vi "ContextHelp_HelpTexts.vi"(0 "HelpText (enum or string)":variant) -> (14 "HelpOut":T2, 15 "NotFound":bool)   [LabVIEW 2014]
uses:
  <resource>/Framework/Providers/Open_GDS/UML/ContextHelp/ContextHelp_ShowType.ctl
  <resource>/Framework/Providers/Open_GDS/UML/ContextHelp/ContextHelp_HelpTexts.ctl
panel:
  in  "HelpText 2":T1
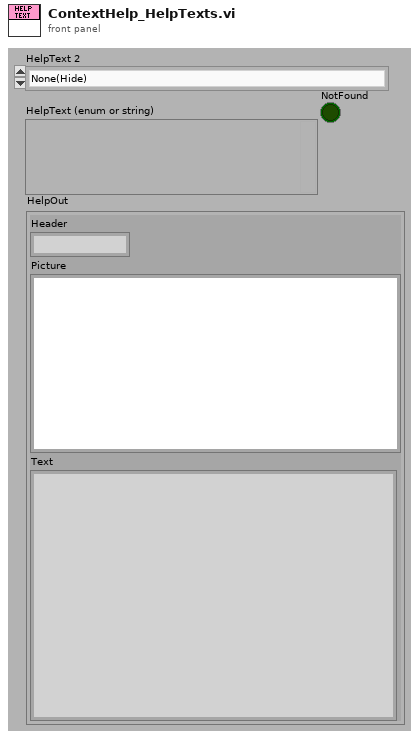
[diagram p1: front panel]
types:
  T1 = typedef "ContextHelp_HelpTexts.ctl" = enum16{"None(Hide)", "Default", "Help", "Welcome", "GettingStarted", "ClassDiagram_Help", "SequenceDiagram_Help", "UseCaseDiagram_Help", "BSelect", "BClass", "BInterface", "BPackage", "BNote", "BDependency", "BInheritance", "BInterfaceImplementation", "BAssociation", "BAggregation", "BCompAggregation", "BNoteConnector", "BObject", "BActionBar", "BCall", "BSystem", "BActor", "BUseCase", "BGeneralization", "BIncludes", "BExtends", "BUseCaseDiagramAssociation", "ClassRelationshipEdge editDialog_Bent Style", "ClassRelationshipEdge editDialog_RelationType", "ClassRelationshipEdge editDialog_Reverse association", "ClassRelationshipEdge editDialog_Start label", "ClassRelationshipEdge editDialog_Middle label", "ClassRelationshipEdge editDialog_End label", "UMLEditor reversedEngineering_Pathes", "ReversedEngineering StateReverseDialog_Help", "ReversedEngineering StateQueuedSettings_Help", "UMLEditor reversedEngineering_AddTopVIs", "UMLEditor reversedEngineering_AddClasses", "UMLEditor reversedEngineering_AddDirs", "UMLEditor reversedEngineering_Recursively", "UMLEditor reversedEngineering_Remove", "UMLEditor reversedEngineering_ClearList", "UMLEditor reversedEngineering_HideSubAss", "UMLEditor reversedEngineering_CreateTypes", "UMLEditor reversedEngineering_OnlyInheritance", "UMLEditor reversedEngineering_CreateApplication", "UMLEditor reversedEngineering_OK", "UMLEditor reversedEngineering_Cancel", "UMLEditor reversedEngineering_Help", "UMLEditor createWizardScriptFile_ScriptfilePath", "UMLEditor createWizardScriptFile_ClassPath", "UMLEditor createWizardScriptFile_Use", "UMLEditor createWizardScriptFile_PrivateDirName", "UMLEditor createWizardScriptFile_DirAppend", "UMLEditor createWizardScriptFile_Separator Character", "UMLEditor createWizardScriptFile_OK", "UMLEditor createWizardScriptFile_Cancel", "UMLEditor createWizardScriptFile_Help", "ClassNode editDialog_Class Name", "InterfaceNode editDialog_Class Name", "ClassNode editDialog_Attribute", "ClassNode editDialog_Methods", "InterfaceNode editDialog_Methods", "ClassNode editDialog_connection", "InterfaceNode editDialog_connection", "ClassNode editDialog_StereoType", "ClassNode editDialog_ShowAttrib", "ClassNode editDialog_ShowMethods", "ClassNode editDialog_ClassPath", "ClassNode editDialog_AddAttribute", "ClassNode editDialog_AddMethod", "InterfaceNode editDialog_AddMethod", "ClassNode AttributeGuide_AttributeName", "ClassNode AttributeGuide_Array?", "ClassNode AttributeGuide_Data Type", "ClassNode AttributeGuide_RefName", "ClassNode AttributeGuide_Preview", "ClassNode AttributeGuide_OK", "ClassNode AttributeGuide_Cancel", "ClassNode MethodGuide_Visibility", "ClassNode MethodGuide_Method Name", "ClassNode MethodGuide_Preview", "ClassNode MethodGuide_OK", "ClassNode MethodGuide_Cancel", "CallNode EditCallProperties_AllButtons", "ObjectNode EditObjectlProperties_AllButtons", "ActorNode EditActorProperties_AllButtons", "UseCaseRelationshipNode EditUseCaselProperties_AllButtons", "UseCaseNode EditUseCaselProperties_AllButtons", "SystemNode EditSystemProperties_AllButtons", "ReversedEngineering UpdateAttributes_AllButtons", "StateNode editDialog_AllButtons", "StateTransition editDialog_AllButtons", "ArrangeNodes Main_Picture", "ArrangeNodes Main_Zoom", "ArrangeNodes Main_Auto Zoom", "ArrangeNodes Main_shorten", "ArrangeNodes Main_Min Length", "ArrangeNodes Main_Max Length", "ArrangeNodes Main_increase", "ArrangeNodes Main_decrease", "ArrangeNodes Main_Shake", "ArrangeNodes Main", "BState", "BInitialState", "BFinalState", "BStateTransition", "StateDiagram_Help", "StateDiagram_PropertiesAllButtons", "ReversedEngineering StateReverseDialog_ClearStates", "ReversedEngineering StateReverseDialog_UseQueuedStateMachines", "ReversedEngineering StateReverseDialog_QueuedSettings", "ReversedEngineering StateReverseDialog_SearchForVIs", "ReversedEngineering StateReverseDialog_SearchCriteria", "OptionsDialog_ClassBasePath", "OptionsDialog_VIPath", "OptionsDialog_ApplicationPath", "OptionsDialog_WizDir", "OptionsDialog_IniFilePath", "OptionsDialog_DefineColors", "OptionsDialog_Help", "OptionsDialog_CreateTypes", "ClassRelationshipEdge editDialog_SplitWire"}
  T2 = typedef "ContextHelp_ShowType.ctl" = cluster{"Header":string, "Picture":picture, "Text":string}
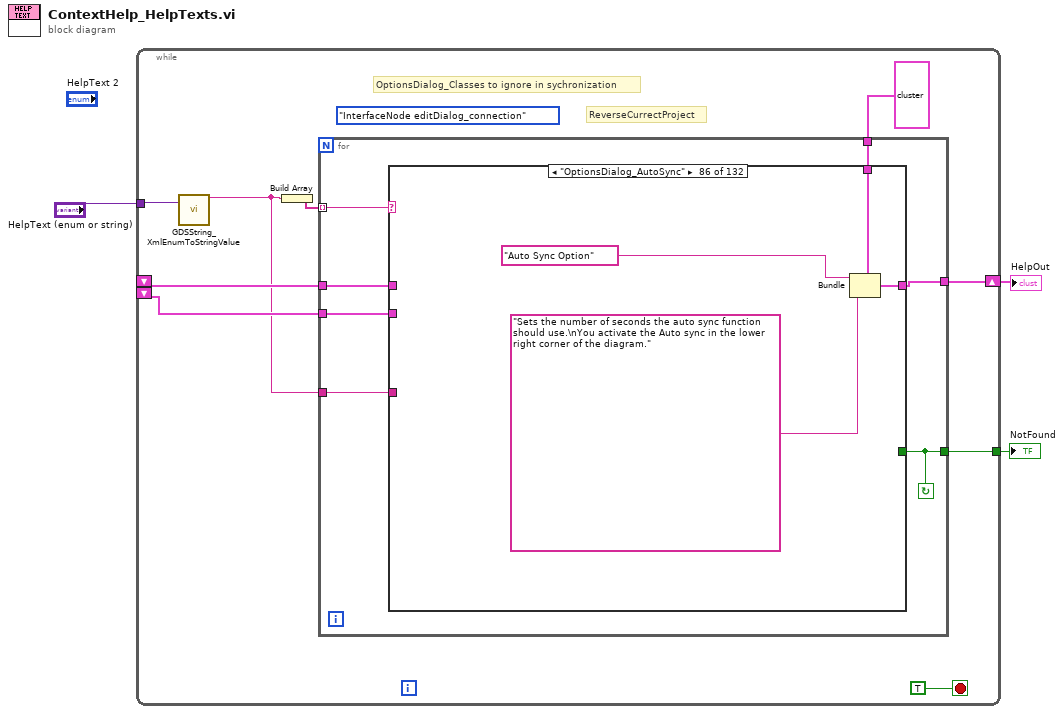
[diagram p0: block diagram]
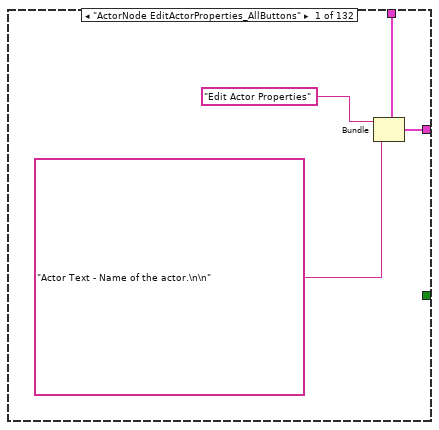
[diagram p2: hidden frame]
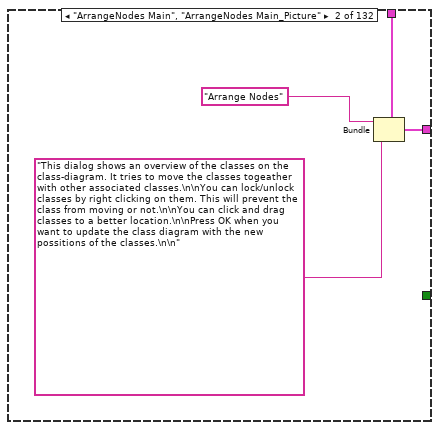
[diagram p3: hidden frame]
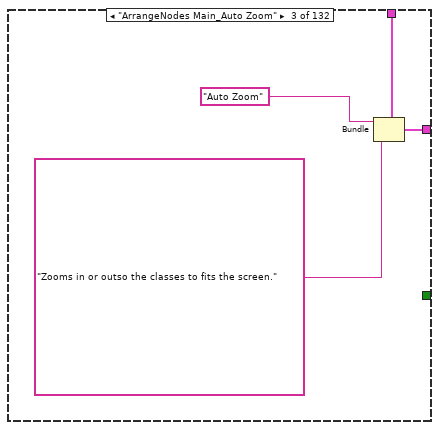
[diagram p4: hidden frame]
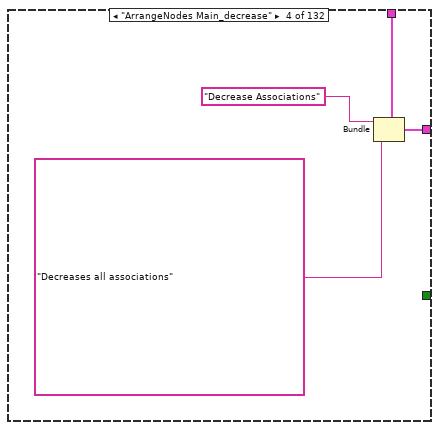
[diagram p5: hidden frame]
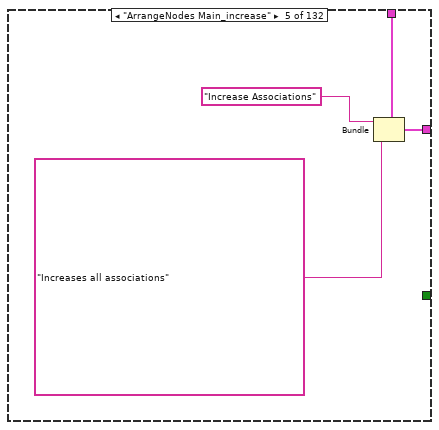
[diagram p6: hidden frame]
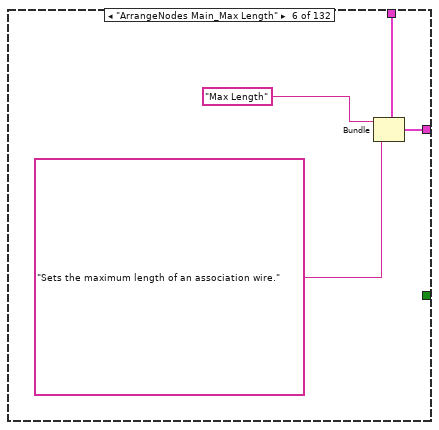
[diagram p7: hidden frame]
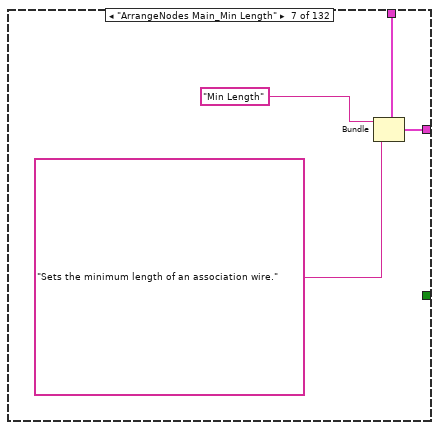
[diagram p8: hidden frame]
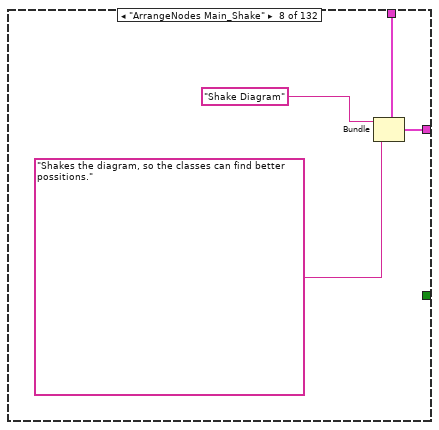
[diagram p9: hidden frame]
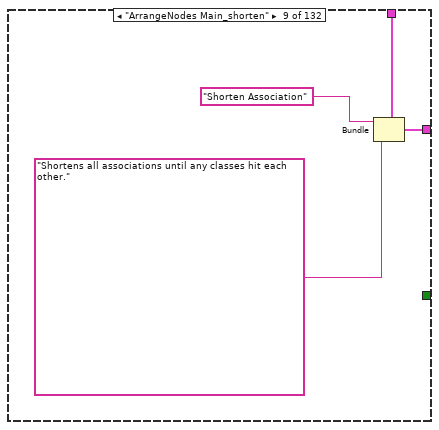
[diagram p10: hidden frame]
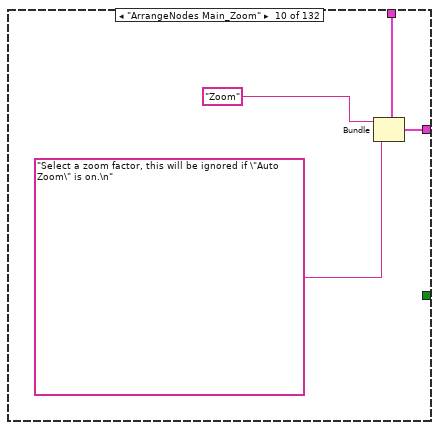
[diagram p11: hidden frame]
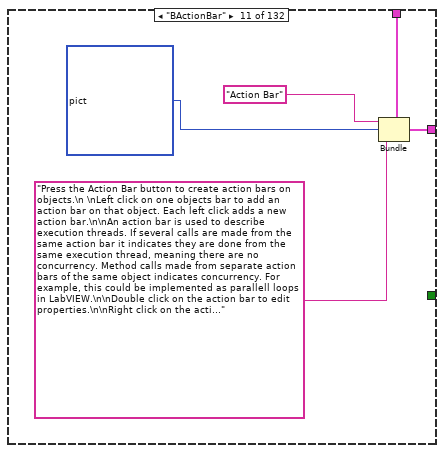
[diagram p12: hidden frame]
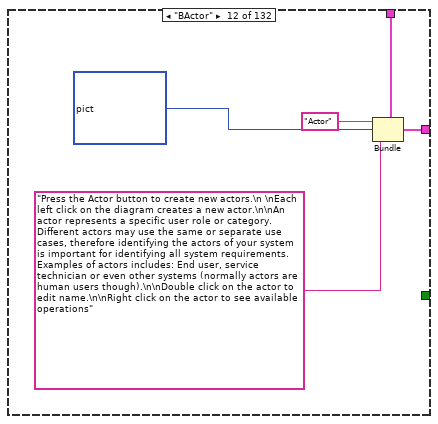
[diagram p13: hidden frame]
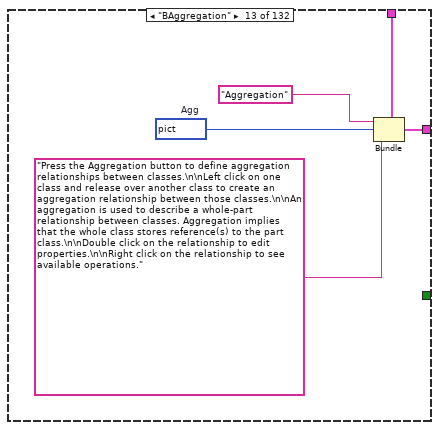
[diagram p14: hidden frame]
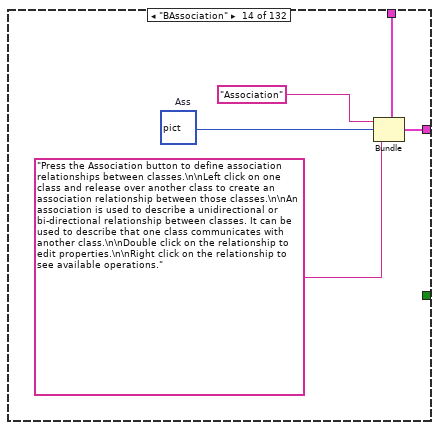
[diagram p15: hidden frame]
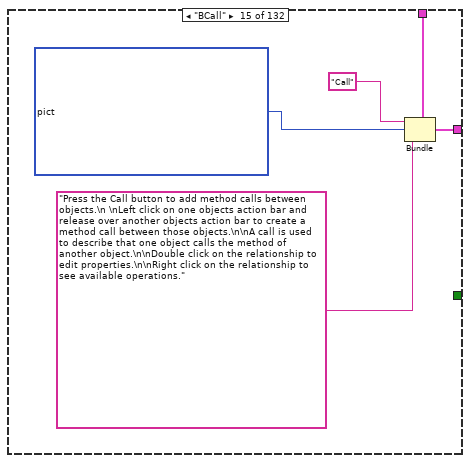
[diagram p16: hidden frame]
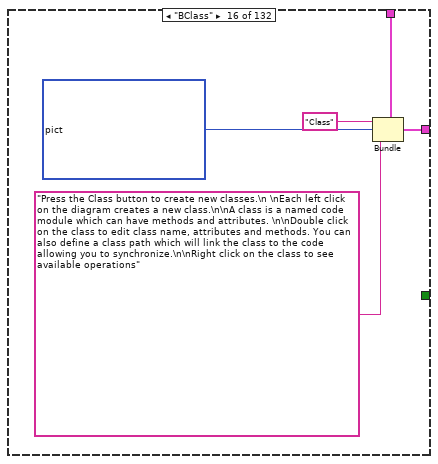
[diagram p17: hidden frame]
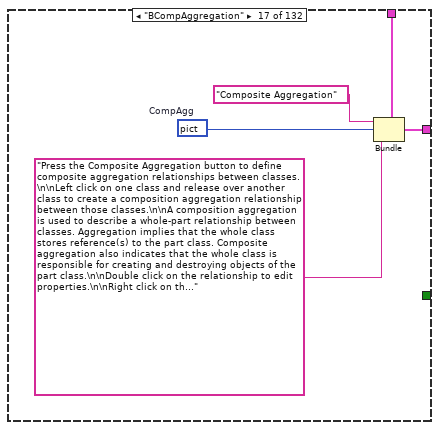
[diagram p18: hidden frame]
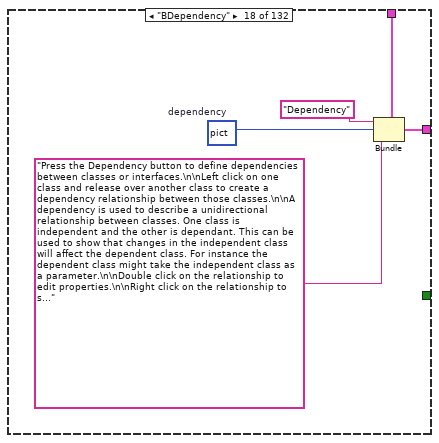
[diagram p19: hidden frame]
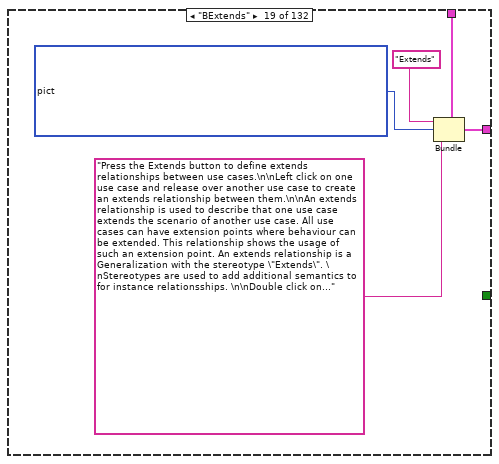
[diagram p20: hidden frame]
diagram:
  n1 = while {
    tunnel: "HelpText (enum or string)" -> [w7]
    shift-right: [w10] -> w2
    shift-left: _ -> [w9]
    shift-left: _ -> [w8]
    tunnel: [w6] -> w1
    stop <- TRUE stop-if-true
    (unwired) ContextHelp_HelpTexts."InterfaceNode editDialog_connection" ("HelpText 2")
    # "OptionsDialog_Classes to ignore in sychronization"
    # "ReverseCurrectProject"
    n2 = call <resource>:"GDSString_XmlEnumToStringValue.vi"("EnumVariantIn(used if String is Empty)"=w7) -> ("EnumValueOut(string)"=w5:string)  [unwired: 2 in, 16 out]
    n3 = Build Array(w5) -> (w4:string[])
    n4 = for {
      tunnel: cluster{string, "empty picture":picture, string} {"", "empty picture"=bytes[0], ""} -> [w19]
      tunnel: [w18] -> w10
      tunnel: w9 -> [w17]
      tunnel: w8 -> [w16]
      tunnel: w5 -> [w13]
      tunnel: [w15] -> w6
      tunnel: w4 -> [w14] mode=indexing
      stop <- w15 continue-if-true
      n5 = case shown="\"OptionsDialog_AutoSync\"" w14 {
        selector: w14 -> [_ _ _ _ _ _ _ _ _ _ _ _ _ _ _ _ _ _ _ _ _ _ _ _ _ _ _ _ _ _ _ _ _ _ _ _ _ _ _ _ _ _ _ _ _ _ _ _ _ _ _ _ _ _ _ _ _ _ _ _ _ _ _ _ _ _ _ _ _ _ _ _ _ _ _ _ _ _ _ _ _ _ _ _ _ _ _ _ _ _ _ _ _ _ _ _ _ _ _ _ _ _ _ _ _ _ _ _ _ _ _ _ _ _ _ _ _ _ _ _ w547 _ _ _ _ _ _ _ _ _ _ _]
        tunnel: [w21 w25 w29 w33 w37 w41 w45 w49 w53 w57 w62 w67 w72 w77 w82 w87 w92 w97 w102 w106 w111 w116 w121 w125 w130 w135 w140 w145 w150 w155 w159 w163 w167 w172 w177 w182 w186 w190 w194 w198 w202 w206 w210 w214 w218 w222 w226 w230 w234 w238 w242 w246 w250 w254 w258 w262 w266 w270 w274 w278 w282 w287 w292 w296 w301 w320 w331 w334 w338 cluster{string, "empty picture":picture, string} {"", "empty picture"=bytes[0], ""} w343 w347 w351 w355 w359 w363 w367 w372 w376 w380 w385 w389 w393 w397 w401 w405 w409 w413 w418 w421 w427 w430 w434 w438 w442 w446 w451 w455 w459 w463 w467 w471 w475 w479 w483 w487 w491 w495 w499 w503 w507 w511 w516 w520 w524 w528 w531 w536 w539 w543 w550 w557 w561 w565 w570 w574 w578 w581 w585 w589 w593 _] -> w18
        tunnel: w19 -> [w20 w24 w28 w32 w36 w40 w44 w48 w52 w56 w61 w66 w71 w76 w81 w86 w91 w96 w101 w105 w110 w115 w120 w124 w129 w134 w139 w144 w149 w154 w158 w162 w166 w171 w176 w181 w185 w189 w193 w197 w201 w205 w209 w213 w217 w221 w225 w229 w233 w237 w241 w245 w249 w253 w257 w261 w265 w269 w273 w277 w281 w286 w291 w295 w300 w319 w330 w333 w337 _ w342 w346 w350 w354 w358 w362 w366 w371 w375 w379 w384 w388 w392 w396 w400 w404 w408 w412 w417 w422 w426 w431 w435 w439 w441 w445 w450 w454 w458 w462 w466 w470 w474 w478 w482 w486 w490 w494 w498 w502 w506 w510 w515 w519 w523 w527 w530 w535 w538 w542 w549 w556 w560 w564 w569 w573 w577 w580 w584 w588 w592 _]
        tunnel: w17 -> [_ _ _ _ _ _ _ _ _ _ _ _ _ _ _ _ _ _ _ _ _ _ _ _ _ _ _ _ _ _ _ _ _ _ _ _ _ _ _ _ _ _ _ _ _ _ _ _ _ _ _ _ _ _ _ _ _ _ _ _ _ _ _ _ _ w315 _ _ _ _ _ _ _ _ _ _ _ _ _ _ _ _ _ _ _ _ _ _ _ _ _ _ _ _ _ _ _ _ _ _ _ _ _ _ _ _ _ _ _ _ _ _ _ _ _ _ _ _ _ _ _ _ _ _ _ _ _ _ _ _ _ _]
        tunnel: w16 -> [_ _ _ _ _ _ _ _ _ _ _ _ _ _ _ _ _ _ _ _ _ _ _ _ _ _ _ _ _ _ _ _ _ _ _ _ _ _ _ _ _ _ _ _ _ _ _ _ _ _ _ _ _ _ _ _ _ _ _ _ _ _ _ _ _ w316 _ _ _ _ _ _ _ _ _ _ _ _ _ _ _ _ _ _ _ _ _ _ _ _ _ _ _ _ _ _ _ _ _ _ _ _ _ _ _ _ _ _ _ _ _ _ _ _ _ _ _ _ _ _ _ _ _ _ _ _ _ _ _ _ _ _]
        tunnel: w13 -> [_ _ _ _ _ _ _ _ _ _ _ _ _ _ _ _ _ _ _ _ _ _ _ _ _ _ _ _ _ _ _ _ _ _ _ _ _ _ _ _ _ _ _ _ _ _ _ _ _ _ _ _ _ _ _ _ _ _ _ _ _ _ _ _ _ w305 _ _ _ _ _ _ _ _ _ _ _ _ _ _ _ _ _ _ _ _ _ _ _ _ _ _ _ _ _ _ _ _ _ _ _ _ _ _ _ _ _ _ _ _ _ _ _ _ _ _ _ _ _ _ _ _ _ _ _ _ _ _ _ _ _ _]
        tunnel: [_ _ _ _ _ _ _ _ _ _ _ _ _ _ _ _ _ _ _ _ _ _ _ _ _ _ _ _ _ _ _ _ _ _ _ _ _ _ _ _ _ _ _ _ _ _ _ _ _ _ _ _ _ _ _ _ _ _ _ _ _ _ _ _ _ _ _ _ _ _ _ _ _ _ _ _ _ _ _ _ _ _ _ _ _ _ _ _ _ _ _ _ _ _ _ _ _ _ _ _ _ _ _ _ _ _ _ _ _ _ _ _ _ _ _ _ _ _ _ _ _ _ _ _ _ _ _ _ _ _ _ TRUE] -> w15
        frame "ActorNode EditActorProperties_AllButtons" {
          n6 = Bundle(cluster=w20, "Edit Actor Properties", "Actor Text - Name of the actor.\n\n") -> (w21:cluster{string, "empty picture":picture, string})  [unwired: 1 out]
        }
        frame "ArrangeNodes Main", "ArrangeNodes Main_Picture" {
          n7 = Bundle(cluster=w24, "Arrange Nodes", "This dialog shows an overview of the classes on the class-diagram. It tries to move the classes togeather with other associated classes.\n\nYou can lock/unlock classes by right clicking on them. This will prevent the class from moving or not.\n\nYou can click and drag classes to a better location.\n\nPress OK when you want to update the class diagram with the new possitions of the classes.\n\n") -> (w25:cluster{string, "empty picture":picture, string})  [unwired: 1 out]
        }
        frame "ArrangeNodes Main_Auto Zoom" {
          n8 = Bundle(cluster=w28, "Auto Zoom", "Zooms in or outso the classes to fits the screen.") -> (w29:cluster{string, "empty picture":picture, string})  [unwired: 1 out]
        }
        frame "ArrangeNodes Main_decrease" {
          n9 = Bundle(cluster=w32, "Decrease Associations", "Decreases all associations") -> (w33:cluster{string, "empty picture":picture, string})  [unwired: 1 out]
        }
        frame "ArrangeNodes Main_increase" {
          n10 = Bundle(cluster=w36, "Increase Associations", "Increases all associations") -> (w37:cluster{string, "empty picture":picture, string})  [unwired: 1 out]
        }
        frame "ArrangeNodes Main_Max Length" {
          n11 = Bundle(cluster=w40, "Max Length", "Sets the maximum length of an association wire.") -> (w41:cluster{string, "empty picture":picture, string})  [unwired: 1 out]
        }
        frame "ArrangeNodes Main_Min Length" {
          n12 = Bundle(cluster=w44, "Min Length", "Sets the minimum length of an association wire.") -> (w45:cluster{string, "empty picture":picture, string})  [unwired: 1 out]
        }
        frame "ArrangeNodes Main_Shake" {
          n13 = Bundle(cluster=w48, "Shake Diagram", "Shakes the diagram, so the classes can find better possitions.") -> (w49:cluster{string, "empty picture":picture, string})  [unwired: 1 out]
        }
        frame "ArrangeNodes Main_shorten" {
          n14 = Bundle(cluster=w52, "Shorten Association", "Shortens all associations until any classes hit each other.") -> (w53:cluster{string, "empty picture":picture, string})  [unwired: 1 out]
        }
        frame "ArrangeNodes Main_Zoom" {
          n15 = Bundle(cluster=w56, "Zoom", "Select a zoom factor, this will be ignored if \"Auto Zoom\" is on.\n") -> (w57:cluster{string, "empty picture":picture, string})  [unwired: 1 out]
        }
        frame "BActionBar" {
          n16 = Bundle(cluster=w61, "Action Bar", "empty picture"=picture bytes[55444] ("Picture"), "Press the Action Bar button to create action bars on objects.\n \nLeft click on one objects bar to add an action bar on that object. Each left click adds a new action bar.\n\nAn action bar is used to describe execution threads. If several calls are made from the same action bar it indicates they are done from the same execution thread, meaning there are no concurrency. Method calls made from separate action bars of the same object indicates concurrency. For example, this could be implemented as parallell loops in LabVIEW.\n\nDouble click on the action bar to edit properties.\n\nRight click on the action bar to see available operations.") -> (w62:cluster{string, "empty picture":picture, string})
        }
        frame "BActor" {
          n17 = Bundle(cluster=w66, "Actor", "empty picture"=picture bytes[33570] ("Picture"), "Press the Actor button to create new actors.\n \nEach left click on the diagram creates a new actor.\n\nAn actor represents a specific user role or category. Different actors may use the same or separate use cases, therefore identifying the actors of your system is important for identifying all system requirements. Examples of actors includes: End user, service technician or even other systems (normally actors are human users though).\n\nDouble click on the actor to edit name.\n\nRight click on the actor to see available operations") -> (w67:cluster{string, "empty picture":picture, string})
        }
        frame "BAggregation" {
          w70 = picture bytes[16480]  # Agg
          n18 = Bundle(cluster=w71, "Aggregation", "empty picture"=w70, "Press the Aggregation button to define aggregation relationships between classes.\n\nLeft click on one class and release over another class to create an aggregation relationship between those classes.\n\nAn aggregation is used to describe a whole-part relationship between classes. Aggregation implies that the whole class stores reference(s) to the part class.\n\nDouble click on the relationship to edit properties.\n\nRight click on the relationship to see available operations.") -> (w72:cluster{string, "empty picture":picture, string})
        }
        frame "BAssociation" {
          w75 = picture bytes[16480]  # Ass
          n19 = Bundle(cluster=w76, "Association", "empty picture"=w75, "Press the Association button to define association relationships between classes.\n\nLeft click on one class and release over another class to create an association relationship between those classes.\n\nAn association is used to describe a unidirectional or bi-directional relationship between classes. It can be used to describe that one class communicates with another class.\n\nDouble click on the relationship to edit properties.\n\nRight click on the relationship to see available operations.") -> (w77:cluster{string, "empty picture":picture, string})
        }
        frame "BCall" {
          n20 = Bundle(cluster=w81, "Call", "empty picture"=picture bytes[165420] ("Picture"), "Press the Call button to add method calls between objects.\n \nLeft click on one objects action bar and release over another objects action bar to create a method call between those objects.\n\nA call is used to describe that one object calls the method of another object.\n\nDouble click on the relationship to edit properties.\n\nRight click on the relationship to see available operations.") -> (w82:cluster{string, "empty picture":picture, string})
        }
        frame "BClass" {
          n21 = Bundle(cluster=w86, "Class", "empty picture"=picture bytes[18080] ("Picture"), "Press the Class button to create new classes.\n \nEach left click on the diagram creates a new class.\n\nA class is a named code module which can have methods and attributes. \n\nDouble click on the class to edit class name, attributes and methods. You can also define a class path which will link the class to the code allowing you to synchronize.\n\nRight click on the class to see available operations") -> (w87:cluster{string, "empty picture":picture, string})
        }
        frame "BCompAggregation" {
          w90 = picture bytes[16480]  # CompAgg
          n22 = Bundle(cluster=w91, "Composite Aggregation", "empty picture"=w90, "Press the Composite Aggregation button to define composite aggregation relationships between classes.\n\nLeft click on one class and release over another class to create a composition aggregation relationship between those classes.\n\nA composition aggregation is used to describe a whole-part relationship between classes. Aggregation implies that the whole class stores reference(s) to the part class. Composite aggregation also indicates that the whole class is responsible for creating and destroying objects of the part class.\n\nDouble click on the relationship to edit properties.\n\nRight click on the relationship to see available operations.") -> (w92:cluster{string, "empty picture":picture, string})
        }
        frame "BDependency" {
          w95 = picture bytes[16480]  # dependency
          n23 = Bundle(cluster=w96, "Dependency", "empty picture"=w95, "Press the Dependency button to define dependencies between classes or interfaces.\n\nLeft click on one class and release over another class to create a dependency relationship between those classes.\n\nA dependency is used to describe a unidirectional relationship between classes. One class is independent and the other is dependant. This can be used to show that changes in the independent class will affect the dependent class. For instance the dependent class might take the independent class as a parameter.\n\nDouble click on the relationship to edit properties.\n\nRight click on the relationship to see available operations.") -> (w97:cluster{string, "empty picture":picture, string})
        }
        frame "BExtends" {
          n24 = Bundle(cluster=w101, "Extends", "empty picture"=picture bytes[185178] ("Picture"), "Press the Extends button to define extends relationships between use cases.\n\nLeft click on one use case and release over another use case to create an extends relationship between them.\n\nAn extends relationship is used to describe that one use case extends the scenario of another use case. All use cases can have extension points where behaviour can be extended. This relationship shows the usage of such an extension point. An extends relationship is a Generalization with the stereotype \"Extends\". \nStereotypes are used to add additional semantics to for instance relationsships. \n\nDouble click on the relationship to edit properties.\n\nRight click on the relationship to see available operations.") -> (w102:cluster{string, "empty picture":picture, string})
        }
        frame "BFinalState" {
          n25 = Bundle(cluster=w105, "Final State", "Press the Final State button to create a new final state.\n\nEach left click on the diagram creates a new final state.\n\nThe final state is the end point for the state machine. There can be several end states in the same state diagram. Transitions can only be to the final state, not from it.\n\nRight click on the final state to see available operations.") -> (w106:cluster{string, "empty picture":picture, string})  [unwired: 1 out]
        }
        frame "BGeneralization" {
          n26 = Bundle(cluster=w110, "Generalization", "empty picture"=picture bytes[270030] ("Picture"), "Press the Generalization button to define generalization relationships actor to actor or use case to use case.\n\nLeft click on one actor (or use case) and release over another actor (or use case) to create a generalization relationship between them.\n\nA generalization is used to describe variations of generalization reationships. Between actors it shows generalization for classes of actors. Between use cases it shows that a use case is a variation of the scenario of another use case.\n\nDouble click on the relationship to edit properties.\n\nRight click on the relationship to see available operations.") -> (w111:cluster{string, "empty picture":picture, string})
        }
        frame "BIncludes" {
          n27 = Bundle(cluster=w115, "Includes", "empty picture"=picture bytes[201810] ("Picture"), "Press the Includes button to define includes relationships between use cases.\n\nLeft click on one use case and release over another use case to create an includes relationship between them.\n\nA includes relationship is used to describe that one use case includes the scenario of another use case. This can be used to extract common descriptions to avoid duplications between use cases. A includes relationship is a Generalization with the stereotype \"Includes\". \nStereotypes are used to add additional semantics to for instance relationsships. \n\nDouble click on the relationship to edit properties.\n\nRight click on the relationship to see available operations.") -> (w116:cluster{string, "empty picture":picture, string})
        }
        frame "BInheritance" {
          w119 = picture bytes[16480]  # Inheritance
          n28 = Bundle(cluster=w120, "Inheritance", "empty picture"=w119, "Press the Inheritance button to define inheritance between classes.\nLeft click on one class and release over another class to create an inheritance relationship between those classes.\n\nAn inheritance relationship is used to describe that one class inherits methods and attributes from another class. Only public and protected methods and attributes are inherited. \n\nDouble click on the relationship to edit properties.\n\nRight click on the relationship to see available operations.") -> (w121:cluster{string, "empty picture":picture, string})
        }
        frame "BInitialState" {
          n29 = Bundle(cluster=w124, "Initial State", "Press the Initial State button to create a new initial state.\n\nThere can be only one initial state in each state diagram.\n\nThe initial state is the starting point for the state machine. Only one state transition from the initial state is allowed per state diagram. No state transitions are allowed to the initial state.\n\nRight click on the initial state to see available operations.") -> (w125:cluster{string, "empty picture":picture, string})  [unwired: 1 out]
        }
        frame "BInterface" {
          w128 = picture bytes[14880]  # Interface
          n30 = Bundle(cluster=w129, "Interface", "empty picture"=w128, "Press the Interface button to create new interfaces.\n \nEach left click on the diagram creates a new interface.\n\nAn interface is a class with public methods only, no private methods and no attributes. An interface never contains implementations of the methods. A class can inherit methods from an interface and provide an implementation of them. \n\nDouble click on the interface to edit name and methods. \n\nRight click on the interface to see available operations.") -> (w130:cluster{string, "empty picture":picture, string})
        }
        frame "BInterfaceImplementation" {
          n31 = Bundle(cluster=w134, "Interface Implementation", "empty picture"=picture bytes[47610] ("new picture"), "Press the Interface Implementation button to define this relationship between an interface and a class.\n\nLeft click on one class and release over an interface to create this relationship.\n\nAn interface implementation relationship is used to describe that a class implements the methods defined in an interface. \n\nDouble click on the relationship to edit properties.\n\nRight click on the relationship to see available operations.") -> (w135:cluster{string, "empty picture":picture, string})
        }
        frame "BNote" {
          n32 = Bundle(cluster=w139, "Note", "empty picture"=picture bytes[16758] ("new picture"), "Press the Note button to create new notes.\n \nEach left click on the diagram creates a new note.\n\nA Note is used to clarify the meaning of the diagram. Use the note connector to connect the note to an element in the diagram.\n\nDouble click on the Note to edit text and colour.\n\nRight click on the Note to see available operations.") -> (w140:cluster{string, "empty picture":picture, string})
        }
        frame "BNoteConnector" {
          n33 = Bundle(cluster=w144, "Note Connector", "empty picture"=picture bytes[16758] ("new picture"), "Press the Note Connector button to connect the note to a graphical element.\n\nLeft click on the note and release where the note should be connected.\n\nRight click on the relationship to see available operations.") -> (w145:cluster{string, "empty picture":picture, string})
        }
        frame "BObject" {
          w148 = picture bytes[35794]  # Object
          n34 = Bundle(cluster=w149, "Object", "empty picture"=w148, "Press the Object button to create new objects.\n \nEach left click on the diagram creates a new object.\n\nAn object is an instance of a Class and will have the methods and attributes of the class it is instantiated from. \n\nDouble click on the object to edit object name. Use the Call button to add method calls between objects.\n\nRight click on the object to see available operations") -> (w150:cluster{string, "empty picture":picture, string})
        }
        frame "BPackage" {
          n35 = Bundle(cluster=w154, "Package", "empty picture"=picture bytes[17536] ("new picture"), "Press the Package button to create new packages.\n \nEach left click on the diagram creates a new Package.\n\nA Package is a logical grouping of classes and interfaces. To disconnect a class/interface from a package open the class/interface property window and select disconnect from package. To connect a class/interface to a package move the class/interface over the package, then open the property window and select connect to package. \n\nDouble click on the package to edit name and description.\n\nRight click on the package to see available operations.") -> (w155:cluster{string, "empty picture":picture, string})
        }
        frame "BSelect" {
          n36 = Bundle(cluster=w158, "Select tool", "Press the Select button, or press SPACEBAR-key, to switch to select mode.\n\nIn select mode diagram elements can be moved by left clicking on them. \n\nDouble click on diagram elements to view and edit properties.\n\nRight click on diagram elements to see available operations.\n\nTIP: Multiple select of diagram elements is supported. Left click on the diagram and drag-and-release mouse to select multiple elements.\n\nTIP: To increase readability you can move connection point of relationships. Left click on the relationship just outside the border of the diagram element (class etc.) and drag to move the connection point.\n\nTIP. View VI descriptions! Press SHIFT-key and move the mouse over the methods of a class to view the corresponding VI descriptions and icons. Context help must be activated and the class must be linked to the code (open Edit Class Properties and add Class Path).") -> (w159:cluster{string, "empty picture":picture, string})  [unwired: 1 out]
        }
        frame "BState" {
          n37 = Bundle(cluster=w162, "State", "Press the State button to create new states.\n\nEach left click on the diagram creates a new state.\n\nA state is a condition during the life of a system, an object or a VI during which it has specific attribute values, satisfies some condition, performs some action or waits for some event.\n\nDouble click on the state to edit state and actions.\n\nRight click on the state to see available operations.\n") -> (w163:cluster{string, "empty picture":picture, string})  [unwired: 1 out]
        }
        frame "BStateTransition" {
          n38 = Bundle(cluster=w166, "State Transition", "Press the State Transition button to create new state transitions.\n\nLeft click on one state and release over another state to create a state transition between those states.\n\nA state transition is a relationship between two states indicating a state change that will take place if an event occurs during the first state. Each state transition represents an event defined by the user.\n\nDouble click on the state transition to edit event.\n\nRight click on the state to see available operations.") -> (w167:cluster{string, "empty picture":picture, string})  [unwired: 1 out]
        }
        frame "BSystem" {
          n39 = Bundle(cluster=w171, "System", "empty picture"=picture bytes[50728] ("Picture"), "Press the System button to create new systems.\n \nEach left click on the diagram creates a new system.\n\nThe system represents the entire system, software and hardware, on which you want to define use cases. \n\nDouble click on the system to edit name.\n\nRight click on the system to see available operations") -> (w172:cluster{string, "empty picture":picture, string})
        }
        frame "BUseCase" {
          n40 = Bundle(cluster=w176, "Use Case", "empty picture"=picture bytes[29220] ("Picture"), "Press the Use Case button to create new use cases.\n \nEach left click on the diagram creates a new use case. Click inside a System to attach use cases to a specific system. Use cases can also be disconnected from a  system. Edit use case properties to disconnect.\n\nA use case defines a specific scenario for using the system. A use case can be described as a sequence of events. If apropriate, the sequence diagram can be used to describe a sequence of interaction between the user and system. In that case the method calls in the sequence diagrams should be interpreted as high level events which does not necessarily correspond with methods on classes.\n\nDouble click on the use case to edit name and connect/disconnect from system.\n\nRight click on the use case to see available operations") -> (w177:cluster{string, "empty picture":picture, string})
        }
        frame "BUseCaseDiagramAssociation" {
          n41 = Bundle(cluster=w181, "Association", "empty picture"=picture bytes[121794] ("Picture"), "Press the Association button to define association relationships between actors and use cases.\n\nLeft click on one actor and release over another use case to create an association relationship between them.\n\nAn association is used to describe the communication between an actor and the system when the use cases is executed. It is a bi-directional relationship since there is normally an interaction between actor and  system.\n\nDouble click on the relationship to edit properties.\n\nRight click on the relationship to see available operations.") -> (w182:cluster{string, "empty picture":picture, string})
        }
        frame "CallNode EditCallProperties_AllButtons" {
          n42 = Bundle(cluster=w185, "Edit Call Properties", "Call text - Name of the method which is called. Potentially parameters can be added.\nExample Call text: \"SetFrequency(100)\"\n\nIs signal - TRUE indicates this is an asynchronous call, meaning the caller will not wait for this method to complete execution. FALSE indicates a synchronous method call.") -> (w186:cluster{string, "empty picture":picture, string})  [unwired: 1 out]
        }
        frame "ClassDiagram_Help" {
          n43 = Bundle(cluster=w189, "Class Diagram", "The Class Diagram displays a static view of all classes and the relationships between them.\n\nSelect desired mouse tool by clicking on the buttons on the top of the window. Use the context help to see the meaning of each mouse tool selection.\n\nRight click or double click on a class to change:\n- class name\n- add/modify attributes\n- add/modify methods\n- browse to the GOOP code of the class (if it exists)\n\nLinking a class to the code makes it possible to synchronize to and from UML on each class. Right click on a class to select synchronization operations.\n\nWhen at least one class is defined the code generation selections are enabled in the Tools menu.\n\nThis diagram can also be created automatically from existing GOOP code. Use the reverse engineer functionality from the Tools menu to do this.\n") -> (w190:cluster{string, "empty picture":picture, string})  [unwired: 1 out]
        }
        frame "ClassNode AttributeGuide_Array?" {
          n44 = Bundle(cluster=w193, "Array?", "Select if the attribute should contain an array of data and in that case the array dimension.") -> (w194:cluster{string, "empty picture":picture, string})  [unwired: 1 out]
        }
        frame "ClassNode AttributeGuide_AttributeName" {
          n45 = Bundle(cluster=w197, "Add Attribute Name", "Attribute name.") -> (w198:cluster{string, "empty picture":picture, string})  [unwired: 1 out]
        }
        frame "ClassNode AttributeGuide_Cancel" {
          n46 = Bundle(cluster=w201, "Cancel", "Press Cancel to exit this dialog without any attribute beeing created.") -> (w202:cluster{string, "empty picture":picture, string})  [unwired: 1 out]
        }
        frame "ClassNode AttributeGuide_Data Type" {
          n47 = Bundle(cluster=w205, "Data Type", "Data type of the current attribute.\n\nFor some selections, like ClassRefNum and TypeRef, an additional text control with show, there class/type name can be entered.") -> (w206:cluster{string, "empty picture":picture, string})  [unwired: 1 out]
        }
        frame "ClassNode AttributeGuide_OK" {
          n48 = Bundle(cluster=w209, "Ok", "Press OK to add the attribute.") -> (w210:cluster{string, "empty picture":picture, string})  [unwired: 1 out]
        }
        frame "ClassNode AttributeGuide_Preview" {
          n49 = Bundle(cluster=w213, "Preview", "Preview of the attribute definition.") -> (w214:cluster{string, "empty picture":picture, string})  [unwired: 1 out]
        }
        frame "ClassNode AttributeGuide_RefName" {
          n50 = Bundle(cluster=w217, "Class/Type Name", "Type definition name or class name.") -> (w218:cluster{string, "empty picture":picture, string})  [unwired: 1 out]
        }
        frame "ClassNode editDialog_AddAttribute" {
          n51 = Bundle(cluster=w221, "Add Attribute Guide", "Click to add a new attribute to the current class.\n\nAttributes can also be added by writing into the text control.") -> (w222:cluster{string, "empty picture":picture, string})  [unwired: 1 out]
        }
        frame "ClassNode editDialog_AddMethod", "InterfaceNode editDialog_AddMethod" {
          n52 = Bundle(cluster=w225, "Add Method Guide", "Click to add a new method to the current class.\n\nMethods can also be added by writing into the text control.") -> (w226:cluster{string, "empty picture":picture, string})  [unwired: 1 out]
        }
        frame "ClassNode editDialog_Attribute" {
          n53 = Bundle(cluster=w229, "Attributes", "Attributes are the data variables of a class.\n\nUse the Add Attribute Guide button to add attributes or simply write in the text control.\n\nAttributes are always private or to be more precise; they are protected. Protected means that they cannot be used from other classes but they can be used from classes inheriting from the current class.") -> (w230:cluster{string, "empty picture":picture, string})  [unwired: 1 out]
        }
        frame "ClassNode editDialog_Class Name" {
          n54 = Bundle(cluster=w233, "Class Name", "Name of the class.") -> (w234:cluster{string, "empty picture":picture, string})  [unwired: 1 out]
        }
        frame "ClassNode editDialog_ClassPath" {
          n55 = Bundle(cluster=w237, "Class Path", "Browse to the source code of this class (if it exists).\nSelect a directory where to store the class-files, llb or the class as files.\nSelect a .ctl file if this class should be a <<TYPE>>/<<ENUM>>, i.e. a LabVIEW Type Def.\nWhen using llb, browse to the directory of the llb file do not select the llb file itself.\n\nThis will enable synchronization on class level to and from UML. \n\nIf context help is enabled class and method desriptions will be read from the source code and displayed in the help window.\n\nRight click on the class to access the synchronization methods.\n\nThere is also a Tools menu selection to synchronize all UML classes from code.") -> (w238:cluster{string, "empty picture":picture, string})  [unwired: 1 out]
        }
        frame "ClassNode editDialog_connection", "InterfaceNode editDialog_connection" {
          n56 = Bundle(cluster=w241, "Connection", "Connects or disconnects this class/interface to a package.") -> (w242:cluster{string, "empty picture":picture, string})  [unwired: 1 out]
        }
        frame "ClassNode editDialog_Methods" {
          n57 = Bundle(cluster=w245, "Methods", "Methods are the VIs of a class.\n\nMethods can have different visibility:\n- Public. Can be used from other classes.\n- Protected. Cannot be used from other classes but can be used by classes inheriting from the current class.\n- Private. Can only be used by methods of the current class.\n\nNOTE. Protected methods are not supported by GOOP. They will be generated as public methods during code generation.") -> (w246:cluster{string, "empty picture":picture, string})  [unwired: 1 out]
        }
        frame "ClassNode editDialog_ShowAttrib" {
          n58 = Bundle(cluster=w249, "Show Attributes?", "Select if the attributes should be visible in the class diagram.") -> (w250:cluster{string, "empty picture":picture, string})  [unwired: 1 out]
        }
        frame "ClassNode editDialog_ShowMethods" {
          n59 = Bundle(cluster=w253, "Show Methods?", "Select if the methods should be visible in the class diagram.") -> (w254:cluster{string, "empty picture":picture, string})  [unwired: 1 out]
        }
        frame "ClassNode editDialog_Stereo Type" {
          n60 = Bundle(cluster=w257, "Stereotype", "Stereotypes are used to describe additional semantics of a class.\n\r\nAvailable choices are:\n- None\n- TYPE\n- ENUM\n- GUI\n- SINGLETON\n- SIGNAL\n- BOUNDARY\n- ENTITY\n- CONTROL\n- LEGACY") -> (w258:cluster{string, "empty picture":picture, string})  [unwired: 1 out]
        }
        frame "ClassNode MethodGuide_Cancel" {
          n61 = Bundle(cluster=w261, "Cancel", "Press Cancel to exit this dialog without any method beeing created.") -> (w262:cluster{string, "empty picture":picture, string})  [unwired: 1 out]
        }
        frame "ClassNode MethodGuide_Method Name" {
          n62 = Bundle(cluster=w265, "Method Name", "Method name") -> (w266:cluster{string, "empty picture":picture, string})  [unwired: 1 out]
        }
        frame "ClassNode MethodGuide_OK" {
          n63 = Bundle(cluster=w269, "OK", "Press OK to add the method.") -> (w270:cluster{string, "empty picture":picture, string})  [unwired: 1 out]
        }
        frame "ClassNode MethodGuide_Preview" {
          n64 = Bundle(cluster=w273, "Preview", "Preview of the method definition.") -> (w274:cluster{string, "empty picture":picture, string})  [unwired: 1 out]
        }
        frame "ClassNode MethodGuide_Visibility" {
          n65 = Bundle(cluster=w277, "Visiblility", "Select visibility for the method.\n\nMethods can have different visibility:\n- Public. Can be used from other classes.\n- Protected. Cannot be used from other classes but can be used by classes inheriting from the current class.\n- Private. Can only be used by methods of the current class.") -> (w278:cluster{string, "empty picture":picture, string})  [unwired: 1 out]
        }
        frame "ClassRelationshipEdge editDialog_Bent Style" {
          n66 = Bundle(cluster=w281, "Bent Styles", "A class relationship could have different \"Bent Styles\", this defines the drawing path of the relationship.\n\nSome times the specified bent style is not possible to use, then an other style is used without changing the bent style properites.\n\nThe styles are:\nSTRAIGHT- no bent is used\nHV- Start horisontal from Start class/node then vertical.\nVH- Vertical/Horisontal\nHVH- Horisontal/Vertical/Horisontal\nVHV- Vertical/Horisontal/Vertical\n") -> (w282:cluster{string, "empty picture":picture, string})  [unwired: 1 out]
        }
        frame "ClassRelationshipEdge editDialog_End label", "ClassRelationshipEdge editDialog_Start label" {
          n67 = Bundle(cluster=w286, "Relationship labels", "empty picture"=picture bytes[55830] ("new picture"), "You can place labels on the relationship to clarify the meaning of the relationship.") -> (w287:cluster{string, "empty picture":picture, string})
        }
        frame "ClassRelationshipEdge editDialog_RelationType" {
          n68 = Bundle(cluster=w291, "Class Relationship Types", "empty picture"=picture bytes[50880] ("new picture"), "Select the type of relationship between the classes/nodes. The availiable types are shown above.\n") -> (w292:cluster{string, "empty picture":picture, string})
        }
        frame "ClassRelationshipEdge editDialog_Reverse association" {
          n69 = Bundle(cluster=w295, "Reverse Relationship/Association", "Swaps the direction of the relationship/association.\nThis could also be done by right-clicking on the association on the diagram.") -> (w296:cluster{string, "empty picture":picture, string})  [unwired: 1 out]
        }
        frame "ClassRelationshipEdge editDialog_SplitWire" {
          n70 = Bundle(cluster=w300, "Relationship settings", "empty picture"=picture bytes[246666] ("new picture"), "If this option is checked the association gets split up. This could be used to avoid getting you diagram hard to read.") -> (w301:cluster{string, "empty picture":picture, string})
        }
        frame "Default", "Help" {
          (unwired) ContextHelp_HelpTexts."Help" ("y")
          w314 = "UML Editor" ("x")
          n71 = Unbundle(w315) -> (w307:string)  [unwired: 2 out]
          n72 = Unbundle(w316) -> (w308:string)  [unwired: 2 out]
          n73 = Equal?(x=w305, y="Help") -> (x = y?=w306:bool)
          n74 = Empty String/Path?(string/path=w307) -> (empty?=w317:bool)
          n75 = Empty String/Path?(string/path=w308) -> (empty?=w318:bool)
          n76 = Equal?(x=w314, y=w307) -> (x = y?=w313:bool)
          n77 = Equal?(x=w314, y=w308) -> (x = y?=w312:bool)
          n78 = Or(x=w313, y=w312) -> (x .or. y?=w309:bool)
          n79 = And(x=w317, y=w318) -> (x .and. y?=w311:bool)
          n80 = Compound Arithmetic op=OR(w309, w311, w306) -> (w310:bool)
          n81 = case shown="True" w310 {
            tunnel: [w321 w327] -> w320
            tunnel: w319 -> [_ w326]
            tunnel: w317 -> [w324 _]
            tunnel: w316 -> [w323 _]
            tunnel: w315 -> [w322 _]
            frame False {
              n82 = Select(t=w323, s=w324, f=w322) -> (s? t:f=w321:cluster{string, "empty picture":picture, string})
            }
            frame True {
              w328 = "To activate online help information, make sure the \"Help->Show Context Help for tools\" is checked, and then just move the mouse over a screen object to get a help text. (This Context help dialog has to be open, and it could be open by pressing the question mark button, or pressing F1).\n\nWhen moving over a class or method while pressing Shift-key, class information will be shown.\nThis is only shown if the class is connect to a class-/control-path."  # To activate online help information, make sure the "Help->Show Context Help for tools" is checked, and then just move the mouse over a screen object to get a help text. (This Context help dialog has to be open, and it could be open by pressing the question mark button, or pressing F1).  When moving over a class or method while pressing Shift-key, class information will be shown. This is only shown if the class is connect to a class-/control-path.
              n83 = Bundle(cluster=w326, "Help window", "empty picture"=picture bytes[12840] ("Picture"), w328) -> (w327:cluster{string, "empty picture":picture, string})
            }
          }
        }
        frame "GettingStarted" {
          n84 = Bundle(cluster=w330, "GettingStarted") -> (w331:cluster{string, "empty picture":picture, string})  [unwired: 2 out]
        }
        frame "InterfaceNode editDialog_Class Name" {
          n85 = Bundle(cluster=w333, "Class Name", "Name of the interface-class.") -> (w334:cluster{string, "empty picture":picture, string})  [unwired: 1 out]
        }
        frame "InterfaceNode editDialog_Methods" {
          n86 = Bundle(cluster=w337, "Methods", "The public methods of the interface.") -> (w338:cluster{string, "empty picture":picture, string})  [unwired: 1 out]
        }
        frame "None(Hide)" {
        }
        frame "ObjectNode EditObjectlProperties_AllButtons" {
          n87 = Bundle(cluster=w342, "Edit Object Properties", "Object Name - Name of the object.\n\nUse a descriptive name.To clarify which class the object is created from the class name can be included in the object name. There are several ways of doing that:\n- If there is only one object from a class the class name can be used as object name.\n- If there are several objects of the same class in the sequence diagram a naming like: \"ObjName : ClassName\" could be used.") -> (w343:cluster{string, "empty picture":picture, string})  [unwired: 1 out]
        }
        frame "OptionsDialog_ApplicationPath" {
          n88 = Bundle(cluster=w346, "Stereotype <<Application>>", "Select the VI to be used as template when generating code for UML classes with stereotype << Application>>") -> (w347:cluster{string, "empty picture":picture, string})  [unwired: 1 out]
        }
        frame "OptionsDialog_Attributes to ignore in sychronization" {
          n89 = Bundle(cluster=w350, "Attributes to ignore in synchronization", "Define string patterns for attributes to be ignored during synchronization and reverse engineering. Normally the default patterns should be sufficient. Since attributes are defined in type defs and type defs are not allowed to be empty (except the lvclass ctl) dummy attributes are used to represent \"no attribute\", the UML tool ignores those attributes since they would clutter the class diagram.") -> (w351:cluster{string, "empty picture":picture, string})  [unwired: 1 out]
        }
        frame "OptionsDialog_Class background color for &lt;&lt;Application/VI&gt;&gt; Stereotypes" {
          n90 = Bundle(cluster=w354, "Class background color for <<Application/VI>> Stereotypes", "Select color for UML classes with stereotype <<Application VI>>. This color will indicate that the UML class represents an application VI rather than a LabVIEW class.") -> (w355:cluster{string, "empty picture":picture, string})  [unwired: 1 out]
        }
        frame "OptionsDialog_Class background color for &lt;&lt;TYPE/ENUM&gt;&gt; Stereotype" {
          n91 = Bundle(cluster=w358, "Class background color for <<TYPE/ENUM>> Stereotype", "Select color for UML class with stereotype <<TYPE>>. This color will indicate that the UML class represents a type definition rather than a LabVIEW class.") -> (w359:cluster{string, "empty picture":picture, string})  [unwired: 1 out]
        }
        frame "OptionsDialog_Class background with path property defined " {
          n92 = Bundle(cluster=w362, "Class background with path property defined ", "Select color for classes with defined path property. This color indicates that your class is connected to code.") -> (w363:cluster{string, "empty picture":picture, string})  [unwired: 1 out]
        }
        frame "OptionsDialog_ClassBasePath" {
          n93 = Bundle(cluster=w366, "Class base path", "Select the root folder to use for connecting the UML classes to code. This folder is used when generating and synchronizing code. The path is used in conjunction with the class folder to create an absolute path for each UML class. By using relative paths the project code can be moved without affecting the code connectivity of existing class diagrams.") -> (w367:cluster{string, "empty picture":picture, string})  [unwired: 1 out]
        }
        frame "OptionsDialog_Classes to ignore in sychronization" {
          n94 = Bundle(cluster=w371, "Classes to ignore in sychronization", "empty picture"=picture bytes[87056] ("new picture"), "Define string patterns for classes to be ignored during synchronization and reverse engineering.\nThis option could be used to hide classes that always are used in your design and just would clutter the class diagram.") -> (w372:cluster{string, "empty picture":picture, string})
        }
        frame "OptionsDialog_CreateTypes" {
          w378 = "Also create dependent types (<<TYPE>>), when synchronizing UML from code."  # Also create dependent types (<<TYPE>>), when synchronizing UML from code.
          n95 = Bundle(cluster=w375, w378, "Check to have UML classes with stereotype <<TYPE>> included for type defs when synchronizing classes") -> (w376:cluster{string, "empty picture":picture, string})  [unwired: 1 out]
        }
        frame "OptionsDialog_Default class background" {
          n96 = Bundle(cluster=w379, "Default class background", "Select default color for UML classes.") -> (w380:cluster{string, "empty picture":picture, string})  [unwired: 1 out]
        }
        frame "OptionsDialog_Help" {
          n97 = Bundle(cluster=w384, "Option Help", "empty picture"=picture bytes[12840] ("Picture"), "Here you can define some global options for the UML Modeller. Move the mouse over the control you like to know more about.") -> (w385:cluster{string, "empty picture":picture, string})
        }
        frame "OptionsDialog_IniFilePath" {
          n98 = Bundle(cluster=w388, "INI-file Path", "This path defines where the UML Modeller ini-file is stored.\nIf the UML Modeller is located on the server you probably would like to have the ini-file locally on your computer.") -> (w389:cluster{string, "empty picture":picture, string})  [unwired: 1 out]
        }
        frame "OptionsDialog_State Background Color" {
          n99 = Bundle(cluster=w392, "State Background Color", "Select background color for states in the state diagram.") -> (w393:cluster{string, "empty picture":picture, string})  [unwired: 1 out]
        }
        frame "OptionsDialog_UseProjectPath" {
          n100 = Bundle(cluster=w396, "Use project file folder as base path for all classes", "Select the root folder to use for connecting the UML classes to code. This folder is used when generating and synchronizing code. The path is used in conjunction with the class folder to create an absolute path for each UML class. By using relative paths the project code can be moved without affecting the code connectivity of existing class diagrams.") -> (w397:cluster{string, "empty picture":picture, string})  [unwired: 1 out]
        }
        frame "OptionsDialog_ActivateUndo", "OptionsDialog_Max number of undo steps" {
          n101 = Bundle(cluster=w400, "Activate the undo function", "Activate and set the maximum undo steps per diagram. The maximum number you can enter is 20. The minimum number you can enter is 4.") -> (w401:cluster{string, "empty picture":picture, string})  [unwired: 1 out]
        }
        frame "OptionsDialog_AutoSync" {
          n102 = Bundle(cluster=w404, "Auto Sync Option", "Sets the number of seconds the auto sync function should use.\nYou activate the Auto sync in the lower right corner of the diagram.") -> (w405:cluster{string, "empty picture":picture, string})  [unwired: 1 out]
        }
        frame "OptionsDialog_VIPath" {
          n103 = Bundle(cluster=w408, "Stereotype <<VI>>", "Select the VI to be used as template when generating code for UML classes with stereotype <<VI>>") -> (w409:cluster{string, "empty picture":picture, string})  [unwired: 1 out]
        }
        frame "OptionsDialog_WizDir" {
          n104 = Bundle(cluster=w412, "Goop Wizard Path", "This path defines where the Goop Wixard is installed.") -> (w413:cluster{string, "empty picture":picture, string})  [unwired: 1 out]
        }
        frame "ReversedEngineering StateQueuedSettings_Help" {
          n105 = Bundle(cluster=w417, "Queued State Machine Settings", "To help the analyse feature for queued state machines some informations is required.\nSelect the VI name (You could use the file-browse button) that perforems the task of taking an array of new states that should be added into the queue of state transitions." ("element")) -> (w418:cluster{string, "empty picture":picture, string})  [unwired: 1 out]
        }
        frame "ReversedEngineering StateReverseDialog_ClearStates" {
          n106 = Bundle(cluster=w422, "Clear All Current States on the diagram", "This option will remove all current states on the diagram before adding the new ones. If not this option is checked only new states will be added." ("element")) -> (w421:cluster{string, "empty picture":picture, string})  [unwired: 1 out]
        }
        frame "ReversedEngineering StateReverseDialog_Help" {
          n107 = Bundle(cluster=w426, "State Diagram Reverse Engineering", "empty picture"=picture bytes[33630] ("Picture"), "Make selections for how the VI state machine will be analyzed.\n\nButton: \"Searching states for actions\" will activate a Sub-VI search in all cases of the state machine. The founded VIs will be stated as action in the state, see picture above.\n\nNOTE. The reverse engineering analysis uses heuristics rather than a complete code analysis to find state transitions. This makes the analysis faster and normally the state machine is correctly displayed but it is not foolproof. \nThis is a description of heuristics used. It is intended as example rather than being a complete list of heuristics (heuristics may change in upgraded versions of the tool):\nFor the event structure - If subscribing for menu item change, the item tags are matched against cases (states) and interpreted as state transitions.\n\nConstants found in a case are matched against cases (states) and interpreted as state transitions.\nArray constants found in a case are matched against cases (states) and interpreted as a list of possible state transitions from the current case. An exception from this rule is if queued state machines are used and the VI inserting a sequence of transitions is found in the case. In this case the list is interpreted as a list of consecutive state transitions between the states in the list.\n" ("element")) -> (w427:cluster{string, "empty picture":picture, string})
        }
        frame "ReversedEngineering StateReverseDialog_QueuedSettings", "ReversedEngineering StateReverseDialog_UseQueuedStateMachines" {
          n108 = Bundle(cluster=w431, "Using Queued Based State Machines", "\"Using Queue Based State Machines\" - In a queue based state machine several events can be generated in each state therefore the state machine analysis are modified to correctly handle this case. A queue based state machine, a.k.a. queued message handler, is formally not a state machine but it is a common and useful design pattern.\n\nTo help the analyse feature for queued state machines some informations is required, use the \"Queue Settings\"-btton to configure these." ("element")) -> (w430:cluster{string, "empty picture":picture, string})  [unwired: 1 out]
        }
        frame "ReversedEngineering StateReverseDialog_SearchCriteria" {
          n109 = Bundle(cluster=w435, "Search states for actions", "\"Limit number of Actions in state (VIs)\"- limits the number of actions (SubVIs), to be added in the state.\n\n\"VI-filter\" combined with \"VI-List\", filter in/out certain VIs, to become actions.\nUse the \"Add...\" buttons to add VIs in the \"VI-list\"-array." ("element")) -> (w434:cluster{string, "empty picture":picture, string})  [unwired: 1 out]
        }
        frame "ReversedEngineering StateReverseDialog_SearchForVIs" {
          n110 = Bundle(cluster=w439, "Search states for actions", "Button: \"Searching states for actions\" will activate a Sub-VI search in all cases of the state machine. The founded VIs will be stated as action in the state.\n\nTo be able to decide which SubVIs, and how many that should be added the option \"Search for Actions(VIs)\" is availible.\nSelect number of actions, and filter in/out certain VIs." ("element")) -> (w438:cluster{string, "empty picture":picture, string})  [unwired: 1 out]
        }
        frame "ReversedEngineering UpdateAttributes_AllButtons" {
          n111 = Bundle(cluster=w441, "Update attributes", "This dialog lets you inspect the modification of the class-attributes. If the attributes looks correct press OK, to replace the old with the new.\n\nUse\" Backup original\", to save the old attributes before applying changes.\n\nPress \"Cancel\" to skip updating the attributes\n\n") -> (w442:cluster{string, "empty picture":picture, string})  [unwired: 1 out]
        }
        frame "SequenceDiagram_Help" {
          n112 = Bundle(cluster=w445, "Sequence Diagram", "The Sequence Diagram displays a dynamic view of the system.\n\nSelect desired mouse tool by clicking on the buttons on the top of the window. Use the context help to see the meaning of each mouse tool selection.\n\nThe sequence diagram is used to show scenarios of interaction between objects.\n\nObjects are shown as vertical bars. Method calls between objects are shown as arrows. Time flows from top to bottom of the diagram. Action bars can be used to show concurrency in the scenarious. See the context help for the Action Bar tool selection for more information.\n\nFirst you need to add objects to be used and give them a name. It is normally a good idea to include the class name in the object name (for instance like this: \"objName : Class Name\") to make it easy to see which class each object is created from.\n\nEach object is represented as a vertical bar.\n\nWhen objects have been added you add an action bar to the object you want to add a method call from. Then select the Call mouse tool to add the method call.\n") -> (w446:cluster{string, "empty picture":picture, string})  [unwired: 1 out]
        }
        frame "StateDiagram_Help" {
          n113 = Bundle(cluster=w450, "State Diagram", "empty picture"=picture bytes[118042] ("Picture"), "State diagrams are used to describe the behavior of a system.  State diagrams describe all of the possible states of an object as events occur.  Each diagram usually represents objects of a single class and track the different states of its objects through the system. \n\nWhen to Use: State Diagrams\nUse state diagrams to demonstrate the behavior of an object through many use cases of the system.  Only use state diagrams for classes where it is necessary to understand the behavior of the object through the entire system.\n\nA state diagram could be connected to a VI (right click on diagram ans select \"Configure\").\nWhen this is done you can right click again and now select \"Update diagram...\", this will analyse the selected VI and draw a state diagram of that state machine found in the VI.\n") -> (w451:cluster{string, "empty picture":picture, string})
        }
        frame "StateDiagram_PropertiesAllButtons" {
          n114 = Bundle(cluster=w454, "Edit State Diagram Properties", "Connect the state diagram to a VI, this will allow reverse engineering.\nMake sure the VI has a state machine on the block diagram.\nRight click on diagram and select \"Update diagram...\".\n") -> (w455:cluster{string, "empty picture":picture, string})  [unwired: 1 out]
        }
        frame "StateNode editDialog_AllButtons" {
          n115 = Bundle(cluster=w458, "Edit State Properties", "State - The name of the state.\nAction - Description of actions performed during this state.") -> (w459:cluster{string, "empty picture":picture, string})  [unwired: 1 out]
        }
        frame "StateTransition editDialog_AllButtons" {
          n116 = Bundle(cluster=w462, "Edit State Transition Properties", "The name of the event.\n\nThe transiton could use different bent style properites.\n\nThe styles are:\nSTRAIGHT- no bent is used\nHV- Start horisontal from Start class/node then vertical.\nVH- Vertical/Horisontal\nHVH- Horisontal/Vertical/Horisontal\nVHV- Vertical/Horisontal/Vertical\nARC- Arc-bent is used\n") -> (w463:cluster{string, "empty picture":picture, string})  [unwired: 1 out]
        }
        frame "SystemNode EditSystemProperties_AllButtons" {
          n117 = Bundle(cluster=w466, "Edit System Properties", "Text - Name or short description of the system.\n\n") -> (w467:cluster{string, "empty picture":picture, string})  [unwired: 1 out]
        }
        frame "UMLEditor createWizardScriptFile__CurrentClassProvider" {
          n118 = Bundle(cluster=w470, "Class provider to use", "Select the class provider to use for the generated classes. All created classes will use the same provider.") -> (w471:cluster{string, "empty picture":picture, string})  [unwired: 1 out]
        }
        frame "UMLEditor createWizardScriptFile_Cancel" {
          n119 = Bundle(cluster=w474, "Cancel", "Press Cancel to exit this dialog without any code beeing generated.") -> (w475:cluster{string, "empty picture":picture, string})  [unwired: 1 out]
        }
        frame "UMLEditor createWizardScriptFile_ClassPath" {
          n120 = Bundle(cluster=w478, "Path for created classes (ignored for classes with a defined class path)", "All classes will be placed in the selected folder. The path defaults to project file path.\nEach class will be created in a separate folder using the class name as folder name plus the optional class folder suffix.") -> (w479:cluster{string, "empty picture":picture, string})  [unwired: 1 out]
        }
        frame "UMLEditor createWizardScriptFile_DirAppend" {
          n121 = Bundle(cluster=w482, "Class folder suffix", "Optional folder name suffix to indicate that the folder contains a class. The suffix is used on all created class folders.") -> (w483:cluster{string, "empty picture":picture, string})  [unwired: 1 out]
        }
        frame "UMLEditor createWizardScriptFile_Help" {
          n122 = Bundle(cluster=w486, "Generate Code from UML", "For each UML class a corresponding lvclass will  be created and added to the selected project. The following items will be generated:\n- Classes.\n- Attributes (data fields)\n- Methods\n- Inheritance\n\nMake sure to select which class provider to use for the generated classes.\n\nTIP 1. After code generation, as well as reverse engineering, each UML class is automatically connected to the lvclass. Now you can right click on the UML class to synchronize minor changes back and forth between UML and code. You can also synchronize the entire diagram by selecting: Tools->Synchronize all classes from code.\n\nTIP 2. You can manually link a UML class to the corresponding code by opening the property window for the UML class and set the property: LVClassPath") -> (w487:cluster{string, "empty picture":picture, string})  [unwired: 1 out]
        }
        frame "UMLEditor createWizardScriptFile_OK" {
          n123 = Bundle(cluster=w490, "OK", "Press OK to start the code generation process.\n\nThis process may take several minutes, depending on the number of classes and methods to be created. ") -> (w491:cluster{string, "empty picture":picture, string})  [unwired: 1 out]
        }
        frame "UMLEditor createWizardScriptFile_PrivateDirName" {
          n124 = Bundle(cluster=w494, "Directories Private Dir Name", "The name of the directory where the private VIs and .ctl-files are placed for each class.\n\nIf directories are selected for class storage, a directory for private files will be created in the class directory.\n\nNormally the default \"Private\" is a good choice to use. Choose one name for the private directory and use it for all classes in your projects. \n\nNOTE. Do not forget to update the properties in the GOOP Wizard so classes created by the GOOP Wizard use the correct name for the private directories.\n") -> (w495:cluster{string, "empty picture":picture, string})  [unwired: 1 out]
        }
        frame "UMLEditor createWizardScriptFile_Project" {
          n125 = Bundle(cluster=w498, "Select project to add classes to", "All created classes will be added to the selected project") -> (w499:cluster{string, "empty picture":picture, string})  [unwired: 1 out]
        }
        frame "UMLEditor createWizardScriptFile_ScriptfilePath" {
          n126 = Bundle(cluster=w502, "Path To Store Script File", "Path to script file.\n\nNormally you do not have to modify this path.\n\nIn the code generation process a script file is created and send to the GOOP Wizard. The script file contains information about all the classes and also all selections made in his UI.") -> (w503:cluster{string, "empty picture":picture, string})  [unwired: 1 out]
        }
        frame "UMLEditor createWizardScriptFile_Separator Character" {
          n127 = Bundle(cluster=w506, "Separator Character", "The separator used between class name and method name in all VIs and .ctl-files of a class.\n\nChoose the suffix to use and ensure all classes in your projects use the same separator.\n\nNOTE. Do not forget to update the properties in the GOOP Wizard so classes created by the GOOP Wizard use the same separator you selected here.\n\nNOTE. The GOOP Wizard will not let you modify the separator on existing classes.  \n\nNOTE. All operating systems (for example Unix) do not work well with spaces in file names. Choosing llb storage would of course eliminate this problem, but you might choose to convert classes stored as llbs to directory storage at a later point. Therefore you should concider this at project start up.\n") -> (w507:cluster{string, "empty picture":picture, string})  [unwired: 1 out]
        }
        frame "UMLEditor createWizardScriptFile_Use" {
          n128 = Bundle(cluster=w510, "Use Directories or LLBs", "Storage selection for classes. Classes can be stored in llb files or as VIs. If the class is stored as VIs a directory will be created for each class.\n\nNOTE. The GOOP Wizard will let you convert classes between llb and directory storage, therefore the selection is reversable.\n\nNOTE. Do not forget to update the properties in the GOOP Wizard so classes created by the GOOP Wizard at a later point use the correct storage.\n\nNOTE. Since this is a property selection in the GOOP Wizard it is conveniant if all classes of your projects are stored either as llb files or VIs, normally you do not mix class storage within a project.\n") -> (w511:cluster{string, "empty picture":picture, string})  [unwired: 1 out]
        }
        frame "UMLEditor reversedEngineering_AddClasses" {
          n129 = Bundle(cluster=w515, "Add (Filter) Classes", "Add classes to analyze. If this selection is used together with top VI it will filter classes used by the top VI." ("element")) -> (w516:cluster{string, "empty picture":picture, string})  [unwired: 1 out]
        }
        frame "UMLEditor reversedEngineering_AddDirs" {
          n130 = Bundle(cluster=w519, "Add (Filter) Directories", "Add directories to be searched. If this selection is used together with top VI it will filter classes used by the top VI. " ("element")) -> (w520:cluster{string, "empty picture":picture, string})  [unwired: 1 out]
        }
        frame "UMLEditor reversedEngineering_AddDirsRec" {
          w525 = "Add (Filter) Directories Recursively"  # Add (Filter) Directories Recursively
          n131 = Bundle(cluster=w523, w525, "Add directories to be searched. If this selection is used together with top VI it will filter classes used by the top VI.\nThis will use a recursive directory search." ("element")) -> (w524:cluster{string, "empty picture":picture, string})  [unwired: 1 out]
        }
        frame "UMLEditor reversedEngineering_AddTopVIs" {
          n132 = Bundle(cluster=w527, "Add Top VIs", "Select a Top VI to start seaching from.\nIf no directories has been added in the list, all found classes will be shown.\nIf any directories has been added in the serach list, only classes within those directories will be analysed." ("element")) -> (w528:cluster{string, "empty picture":picture, string})  [unwired: 1 out]
        }
        frame "UMLEditor reversedEngineering_Cancel" {
          n133 = Bundle(cluster=w530, "Cancel", "Press Cancel to exit this dialog without any UML beeing generated.") -> (w531:cluster{string, "empty picture":picture, string})  [unwired: 1 out]
        }
        frame "UMLEditor reversedEngineering_ClearList" {
          n134 = Bundle(cluster=w535, "Clear list", "Remove all entries in the search list." ("element")) -> (w536:cluster{string, "empty picture":picture, string})  [unwired: 1 out]
        }
        frame "UMLEditor reversedEngineering_CreateApplication" {
          n135 = Bundle(cluster=w538, "Create an application node", "This will place an stereotyped <<APPLICATION>> class, on the diagram that represents the Top-VI. This is actually no class and therefor don't have attributes or methods.") -> (w539:cluster{string, "empty picture":picture, string})  [unwired: 1 out]
        }
        frame "UMLEditor reversedEngineering_CreateTypes" {
          n136 = Bundle(cluster=w542, "Create Types", "Select if types (TypeDefs *.ctl-files) should be included in the class diagram.") -> (w543:cluster{string, "empty picture":picture, string})  [unwired: 1 out]
        }
        frame "UMLEditor reversedEngineering_Help", "UMLEditor reversedEngineering_Pathes" {
          n137 = case shown="Default" w547 {
            tunnel: ["Select files to be reverse engineered.\n\nAdd a top VI to generate a class diagram for an entire application. To generate a class diagram for a subset of the classes within an application the class and directory selections can be used together with a top VI selection. Only selected classes and classes within the selected directories will be included in the class diagram.\n\nIf no top VI is added all selected classes and classes within selected directories will be included in the class diagram." "Reverse Engineering is the process of generating UML class diagram from existing GOOP code.\n\nYou must select what code to generate UML from. If you select the application top VI the entire application will be analyzed. As an alternative you can browse to classes to be analyzed.\n\nThe check box selections lets you affect how the code is analyzed and displayed in the class diagram.\n\nThe reverse engineering process performes an advanced analysis to find different class relationships as well as finding all methods and attributes of each class.\n\nAll the relationships (see the on-line help for each button in the class diagram window) the tool lets you define between classes can also be reverse engineered.\n\nTIP 1. You can activate reverse engineering from the LabVIEW project explorer. Right click on MyComputer->UML->View all classes in class diagram… This feature will open the Reverse Engineering UI with all classes in the project loaded. \nOr alternatively: right click on an individual lvclass: MyClass.lvclass->UML->View class in class diagram. This feature will create a new class diagram with the selected lvclass reverse engineered.\n\nTIP 2. After reverse engineering, as well as code generation, each UML class is automatically connected to the lvclass. Now you can right click on the UML class to synchronize minor changes back and forth between UML and code. You can also synchronize the entire diagram by selecting: Tools->Synchronize all classes from code.\n\nTIP 3. You can manually link a UML class to the corresponding code by opening the property window for the UML class and set the property: LVClassPath\n"] -> w551
            tunnel: ["Top VIs, classes (llbs/dirs) and directories that should be analyzed" "Reverse Engineering"] -> w546
            frame "UMLEditor reversedEngineering_Pathes" {
            }
            frame Default {
            }
          }
          n138 = Bundle(cluster=w549, w546, "empty picture"=picture bytes[429936] ("Picture"), w551) -> (w550:cluster{string, "empty picture":picture, string})
        }
        frame "UMLEditor reversedEngineering_HideSubAss" {
          n139 = Bundle(cluster=w556, "Hide SubClass Assoiciations", "If a base class  already has a relationship with an other class, this class will not show an extra relationship to that class.\n\nExample. A base class aggregates another class. This implies the base class has attribute(s) for holding reference(s) to objects of the other class. These attributes will be inherited by sub classes. Therefore sub classes will also aggregate the other class. By checking this selection only the base class aggregation will be shown in the UML diagram. This is normally the best choice to avoid cluttering the diagram.") -> (w557:cluster{string, "empty picture":picture, string})  [unwired: 1 out]
        }
        frame "UMLEditor reversedEngineering_OK" {
          n140 = Bundle(cluster=w560, "OK", "Press OK to generate UML for the selected classes.\n\nThis process may take several minutes, depending on the number of classes and methods to be analyzed. ") -> (w561:cluster{string, "empty picture":picture, string})  [unwired: 1 out]
        }
        frame "UMLEditor reversedEngineering_OnlyInheritance" {
          n141 = Bundle(cluster=w564, "Only Inheritance Classes", "Select to evaluate this class only and its base-classes, i.e. the inheritance hierarchy.") -> (w565:cluster{string, "empty picture":picture, string})  [unwired: 1 out]
        }
        frame "UMLEditor reversedEngineering_Recursively" {
          n142 = Bundle(cluster=w569, "Add Search directories recursively", "When selecting a filter directory, the directory and all its sub-directories." ("element")) -> (w570:cluster{string, "empty picture":picture, string})  [unwired: 1 out]
        }
        frame "UMLEditor reversedEngineering_Remove" {
          n143 = Bundle(cluster=w573, "Remove", "Remove one entry in search list." ("element")) -> (w574:cluster{string, "empty picture":picture, string})  [unwired: 1 out]
        }
        frame "UMLEditor reversedEngineering_ReverseCurrectProject" {
          n144 = Bundle(cluster=w577, "Add all classes from project", "Add all classes from the current project." ("element")) -> (w578:cluster{string, "empty picture":picture, string})  [unwired: 1 out]
        }
        frame "UseCaseDiagram_Help" {
          n145 = Bundle(cluster=w580, "Use Case Diagram", "The Use Case Diagram shows use cases provided by the system and user categories which are called Actors.\n\nSelect desired mouse tool by clicking on the buttons on the top of the window. Use the context help to see the meaning of each mouse tool selection.\n\nThe use case diagram is used to clarify the system boundaries and show the functionality provided. This diagram is normally used during the requirements phase of development.\n\nThe elements of this diagram are:\n- Use cases. These are user scenarios.\n- Actors. These repesent user categories or roles.\n- System. This lets you define which system that provides (implements) the different use cases.\nSee the context help for more information about these concepts.\n\nFirst add a system to the diagram. This represents the system you are about to build. Then consider if the users of this system have different roles and thus could have different requirements on the system. Add an Actor for each role.\nThen add use cases inside the system. Use the Association relationship to show which actor is using which use case.") -> (w581:cluster{string, "empty picture":picture, string})  [unwired: 1 out]
        }
        frame "UseCaseNode EditUseCaselProperties_AllButtons" {
          n146 = Bundle(cluster=w584, "Edit Use Case Properties", "Use Case text - Name of the use case.\n\nDisconnect From System - Select to disconnect this use case from the system it currently belongs to. This selection is only visible for use cases which belongs to a system.\n\nConnect To System - Select to connect this use case to the system it is currently placed over. This selection is only visible for disconnected use cases which are placed over a system.\n\n") -> (w585:cluster{string, "empty picture":picture, string})  [unwired: 1 out]
        }
        frame "UseCaseRelationshipNode EditUseCaselProperties_AllButtons" {
          n147 = Bundle(cluster=w588, "Edit Actor Properties", "Label - A label can be used to clarify the interaction between actor and use case.\n\n") -> (w589:cluster{string, "empty picture":picture, string})  [unwired: 1 out]
        }
        frame "Welcome" {
          n148 = Bundle(cluster=w592, "Welcome") -> (w593:cluster{string, "empty picture":picture, string})  [unwired: 2 out]
        }
        frame Default {
        }
      }
    }
  }
  "HelpOut" <- w2
  "NotFound" <- w1
